vi "get_x.vi"(0 "HB_Simple":refnum<class "HB_Simple.lvclass">, 5 "error in (no error)":errorcluster) -> (14 "dup HB_Simple":refnum<class "HB_Simple.lvclass">, 16 "x":dbl, 19 "error out":errorcluster)   [LabVIEW 2009, in "HB_BaseClass_Examples.lvlib" / "HB_Simple.lvclass"]
doc: "Read value of x."
uses:
  HB_Simple.lvclass
  HB_Simple.lvclass/HB_Simple.ctl
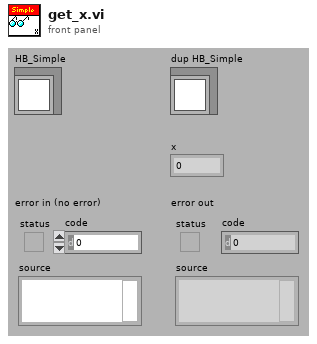
[diagram p1: front panel]
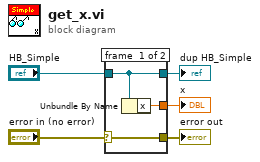
[diagram p0: block diagram]
diagram:
  n1 = case shown="No Error" "error in (no error)" {
    selector: "error in (no error)" -> [w8 w9]
    tunnel: [w8 w9] -> w4
    tunnel: [w7 w10] -> w2
    tunnel: "HB_Simple" -> [w7 w10]
    tunnel: [w6 _] -> w1
    frame #0 {
      n2 = Unbundle By Name(w7) -> ("x"=w6:dbl)
    }
    frame #1 {
    }
  }
  "error out" <- w4
  "dup HB_Simple" <- w2
  "x" <- w1
